vi "sub FM0decodeGet16 v2.vi"(10 "threshold":i32=3, 11 "RN16 waveform":i16[](array[numeric])) -> (3 "RN16 array":i32[](array[numeric]))   [LabVIEW 2015]
doc: "This example shows how the Write to Text File and Read from Text File functions operate using different options."
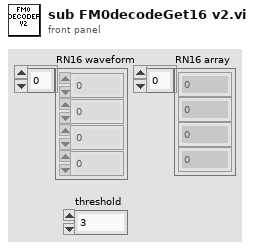
[diagram p1: front panel]
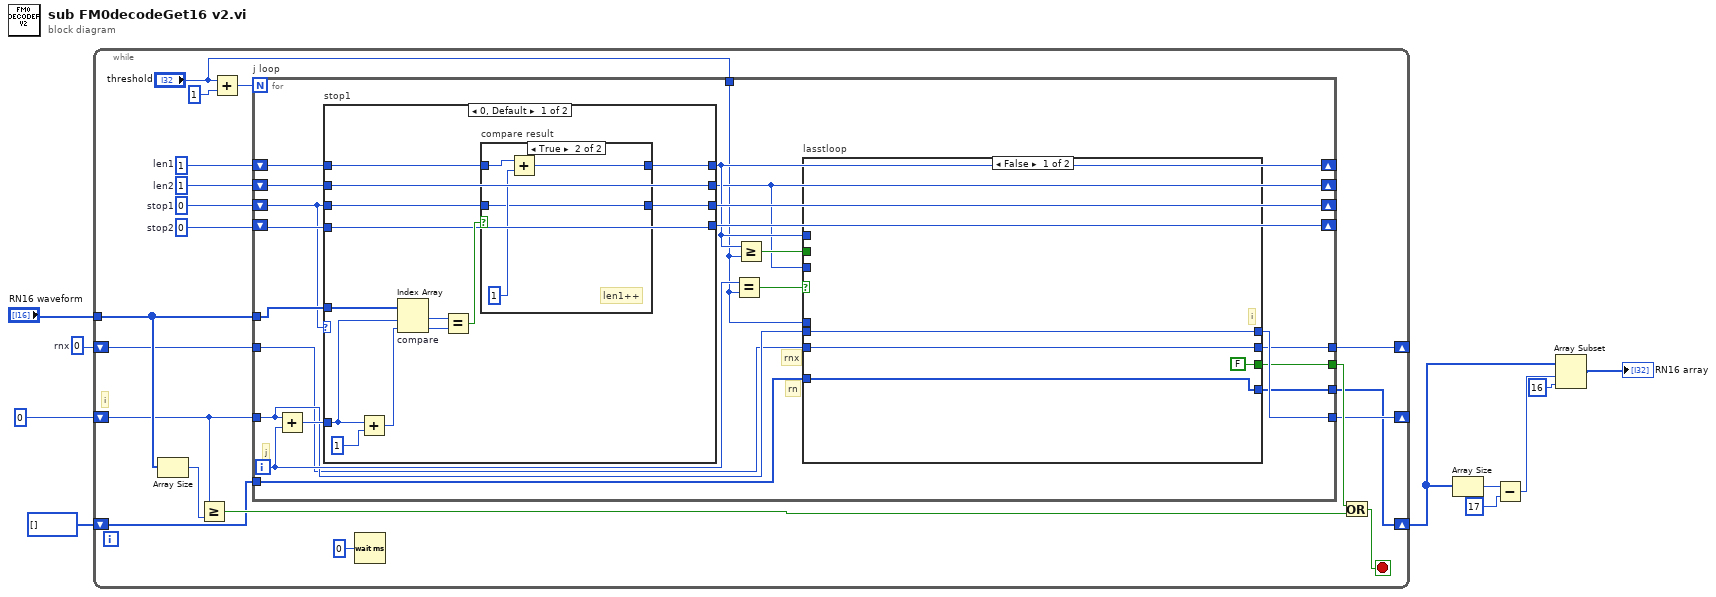
[diagram p0: block diagram]
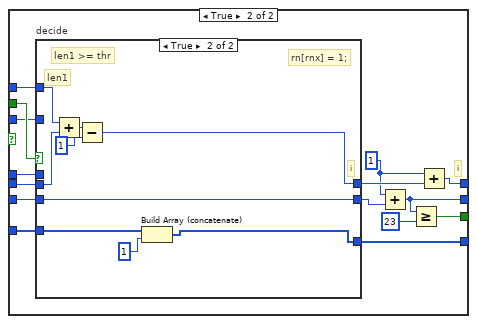
[diagram p2: hidden frame]
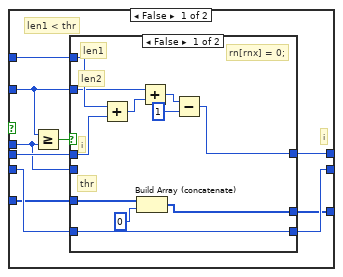
[diagram p3: hidden frame]
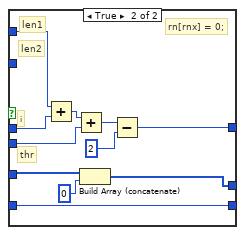
[diagram p4: hidden frame]
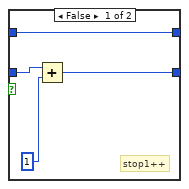
[diagram p5: hidden frame]
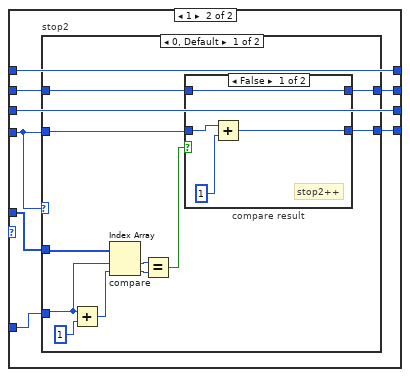
[diagram p6: hidden frame]
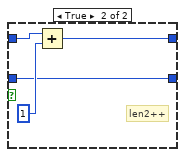
[diagram p7: hidden frame]
diagram:
  w10 = 0  # rnx
  n1 = while {
    tunnel: "RN16 waveform" -> [w25]
    shift-right: [w13] -> _
    shift-left: 0 -> [w14]
    shift-right: [w16] -> _
    shift-left: w10 -> [w15]
    shift-right: [w11] -> w7
    shift-left: i32[] [] -> [w12]
    stop <- w22 stop-if-true
    w29 = 0  # stop2
    w28 = 0  # stop1
    w27 = 1  # len2
    w26 = 1  # len1
    # "i"
    n2 = Array Size(array=w25) -> (size(s)=w24:i32)
    n3 = Greater Or Equal?(x=w14, y=w24) -> (x >= y?=w21:bool)
    n4 = Add(x="threshold", y=1) -> (x+y=w18:i32)
    n5 = for "j loop" {
      N: w18 -> [_]
      tunnel: w25 -> [w46]
      shift-right: [w38] -> _
      shift-left: w26 -> [w50]
      shift-right: [w44] -> _
      shift-left: w28 -> [w45]
      shift-right: [w43] -> _
      shift-left: w29 -> [w48]
      shift-right: [w34] -> _
      shift-left: w27 -> [w49]
      tunnel: "threshold" -> [w32]
      tunnel: [w33] -> w23
      tunnel: w14 -> [w39]
      tunnel: [w37] -> w13
      tunnel: w15 -> [w36]
      tunnel: [w35] -> w16
      tunnel: w12 -> [w31]
      tunnel: [w30] -> w11
      i -> [w42]
      # "rn"
      # "rnx"
      # "j"
      n6 = Add(x=w39, y=w42) -> (x+y=w47:i32)
      n7 = case "stop1" shown="0, Default" w45 {
        tunnel: w50 -> [w116 w139]
        tunnel: w49 -> [w112 w134]
        tunnel: w48 -> [w111 w136]
        tunnel: w47 -> [w122 w132]
        tunnel: w46 -> [w120 w137]
        tunnel: [w115 w139] -> w38
        tunnel: w45 -> [w114 w138]
        tunnel: [w113 w138] -> w44
        tunnel: [w111 w135] -> w43
        tunnel: [w112 w133] -> w34
        frame 0, Default {
          n8 = Add(x=w122, y=1) -> (x+y=w123:i32)
          n9 = Index Array "compare"(array=w120, index #1=w122, index #2=w123) -> (element #1=w118:i16, element #2=w119:i16)
          n10 = Equal?(x=w118, y=w119) -> (x = y?=w117:bool)
          n11 = case "compare result" shown="True" w117 {
            tunnel: w116 -> [w127 w131]
            tunnel: [w127 w130] -> w115
            tunnel: w114 -> [w125 w128]
            tunnel: [w126 w128] -> w113
            frame False {
              # "stop1++"
              n12 = Add(x=w125, y=1) -> (x+y=w126:i32)
            }
            frame True {
              # "len1++"
              n13 = Add(x=w131, y=1) -> (x+y=w130:i32)
            }
          }
        }
        frame 1 {
          n14 = case "stop2" shown="0, Default" w136 {
            tunnel: w137 -> [w147 _]
            tunnel: w136 -> [w146 w159]
            tunnel: [w145 w159] -> w135
            tunnel: w134 -> [w144 w160]
            tunnel: [w143 w160] -> w133
            tunnel: w132 -> [w140 _]
            frame 0, Default {
              n15 = Add(x=w140, y=1) -> (x+y=w148:i32)
              n16 = Index Array "compare"(array=w147, index #1=w140, index #2=w148) -> (element #1=w150:i16, element #2=w149:i16)
              n17 = Equal?(x=w150, y=w149) -> (x = y?=w141:bool)
              n18 = case "compare result" shown="False" w141 {
                tunnel: w144 -> [w154 w158]
                tunnel: [w154 w157] -> w143
                tunnel: w146 -> [w152 w155]
                tunnel: [w153 w155] -> w145
                frame False {
                  # "stop2++"
                  n19 = Add(x=w152, y=1) -> (x+y=w153:i32)
                }
                frame True {
                  # "len2++"
                  n20 = Add(x=w158, y=1) -> (x+y=w157:i32)
                }
              }
            }
            frame 1 {
            }
          }
        }
      }
      n21 = Equal?(x=w42, y=w32) -> (x = y?=w41:bool)
      n22 = Greater Or Equal?(x=w38, y=w32) -> (x >= y?=w40:bool)
      n23 = case "lasstloop" shown="False" w41 {
        tunnel: w40 -> [_ w67]
        tunnel: w39 -> [w54 w69]
        tunnel: w38 -> [_ w68]
        tunnel: [w54 w60] -> w37
        tunnel: w36 -> [w53 w58]
        tunnel: [w53 w65] -> w35
        tunnel: w34 -> [_ w66]
        tunnel: [FALSE w63] -> w33
        tunnel: w32 -> [_ w62]
        tunnel: w31 -> [w51 w56]
        tunnel: [w51 w55] -> w30
        frame False {
          # "i"
        }
        frame True {
          w59 = 1 ("y")
          # "i"
          n24 = case "decide" shown="True" w67 {
            tunnel: w69 -> [w79 w109]
            tunnel: w68 -> [w75 w110]
            tunnel: [w74 w107] -> w61
            tunnel: w66 -> [w77 _]
            tunnel: w62 -> [w76 _]
            tunnel: [w72 w105] -> w57
            tunnel: w58 -> [w73 w105]
            tunnel: w56 -> [w71 w104]
            tunnel: [w70 w103] -> w55
            frame False {
              # "i"
              # "len1 < thr"
              n25 = Greater Or Equal?(x=w77, y=w76) -> (x >= y?=w78:bool)
              n26 = case shown="False" w78 {
                tunnel: w77 -> [w87 _]
                tunnel: w79 -> [w89 w100]
                tunnel: w76 -> [_ w98]
                tunnel: w75 -> [w90 w101]
                tunnel: [w84 w95] -> w74
                tunnel: [w83 w94] -> w72
                tunnel: w73 -> [w83 w94]
                tunnel: w71 -> [w82 w93]
                tunnel: [w80 w92] -> w70
                frame False {
                  # "rn[rnx] = 0;"
                  # "thr"
                  # "len2"
                  # "i"
                  # "len1"
                  n27 = Add(x=w90, y=w89) -> (x+y=w88:i32)
                  n28 = Build Array (concatenate)(w82, 0 ("new element/subarray")) -> (w80:i32[])
                  n29 = Add(x=w87, y=w88) -> (x+y=w86:i32)
                  n30 = Subtract(x=w86, y=1) -> (x-y=w84:i32)
                }
                frame True {
                  # "rn[rnx] = 0;"
                  # "len2"
                  # "thr"
                  # "i"
                  # "len1"
                  n31 = Add(x=w101, y=w100) -> (x+y=w99:i32)
                  n32 = Add(x=w99, y=w98) -> (x+y=w97:i32)
                  n33 = Build Array (concatenate)(w93, 0 ("new element/subarray")) -> (w92:i32[])
                  n34 = Subtract(x=w97, y=2) -> (x-y=w95:i32)
                }
              }
            }
            frame True {
              # "rn[rnx] = 1;"
              # "len1"
              # "i"
              # "len1 >= thr"
              n35 = Add(x=w110, y=w109) -> (x+y=w108:i32)
              n36 = Subtract(x=w108, y=1) -> (x-y=w107:i32)
              n37 = Build Array (concatenate)(w104, 1 ("new element/subarray")) -> (w103:i32[])
            }
          }
          n38 = Add(x=w59, y=w57) -> (x+y=w65:i32)
          n39 = Greater Or Equal?(x=w65, y=23) -> (x >= y?=w63:bool)
          n40 = Add(x=w59, y=w61) -> (x+y=w60:i32)
        }
      }
    }
    n41 = Wait (ms)(milliseconds to wait=u32 0) -> ()  [unwired: 1 out]
    n42 = Or(x=w23, y=w21) -> (x .or. y?=w22:bool)
  }
  n43 = Array Size(array=w7) -> (size(s)=w6:i32)
  n44 = Subtract(x=w6, y=17) -> (x-y=w4:i32)
  n45 = Array Subset(array=w7, index=w4, length=16) -> (→"RN16 array":i32[])
